vi "realTimeDisplay_AS2.vi"() -> ()   [LabVIEW 2016]
uses:
  <userlib>/RSA_API/RSA_API.lvlib
panel:
  in  "Done":bool
  in  "Cluster":T1 {"verticalUnit" items=["SpectrumVerticalUnit_dBm", "SpectrumVerticalUnit_Watt", "SpectrumVerticalUnit_Volt", "SpectrumVerticalUnit_Amp", "SpectrumVerticalUnit_dBmV"]; "window" items=["SpectrumWindow_Kaiser", "SpectrumWindow_Mil6dB", "SpectrumWindow_BlackmanHarris", "SpectrumWindow_Rectangle", "SpectrumWindow_FlatTop", "SpectrumWindow_Hann"]}
  in  "center freq":dbl
  in  "refLevel in":dbl
  in  "Trace number":u32(ring) items=["SpectrumTrace1", "SpectrumTrace2", "SpectrumTrace3"]
  out "traceData out":sgl[](graph)
  out "outTracePoints out":i32
  out "Trace Ready":bool
  out "enable out":bool
  out "refLevel out":dbl
  out "cf out":dbl
  in  "deviceID":i32
  out "deviceType out":string
  out "deviceSerial out":string
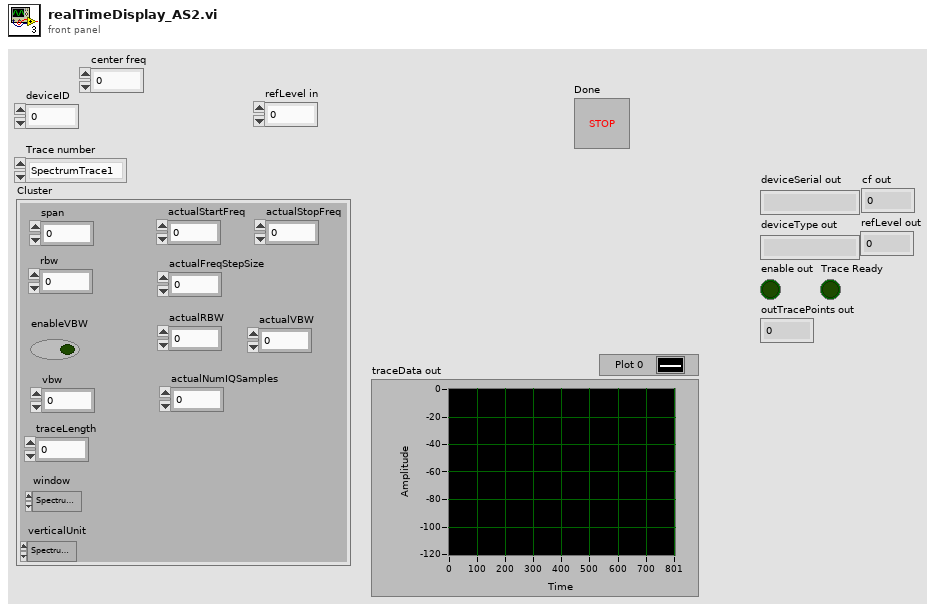
[diagram p1: front panel]
types:
  T1 = cluster{"span":dbl, "rbw":dbl, "enableVBW":bool, "vbw":dbl, "traceLength":i32, "window":u32, "verticalUnit":u32, "actualStartFreq":dbl, "actualStopFreq":dbl, "actualFreqStepSize":dbl, "actualRBW":dbl, "actualVBW":dbl, "actualNumIQSamples":i32}
  T2 = cluster{"span":dbl, "rbw":dbl, "enableVBW":bool, "vbw":dbl, "traceLength":i32, "window":u32, "verticalUnit":u32, dbl, dbl, "actualFreqStepSize":dbl, "actualRBW":dbl, "actualVBW":dbl, "actualNumIQSamples":i32}
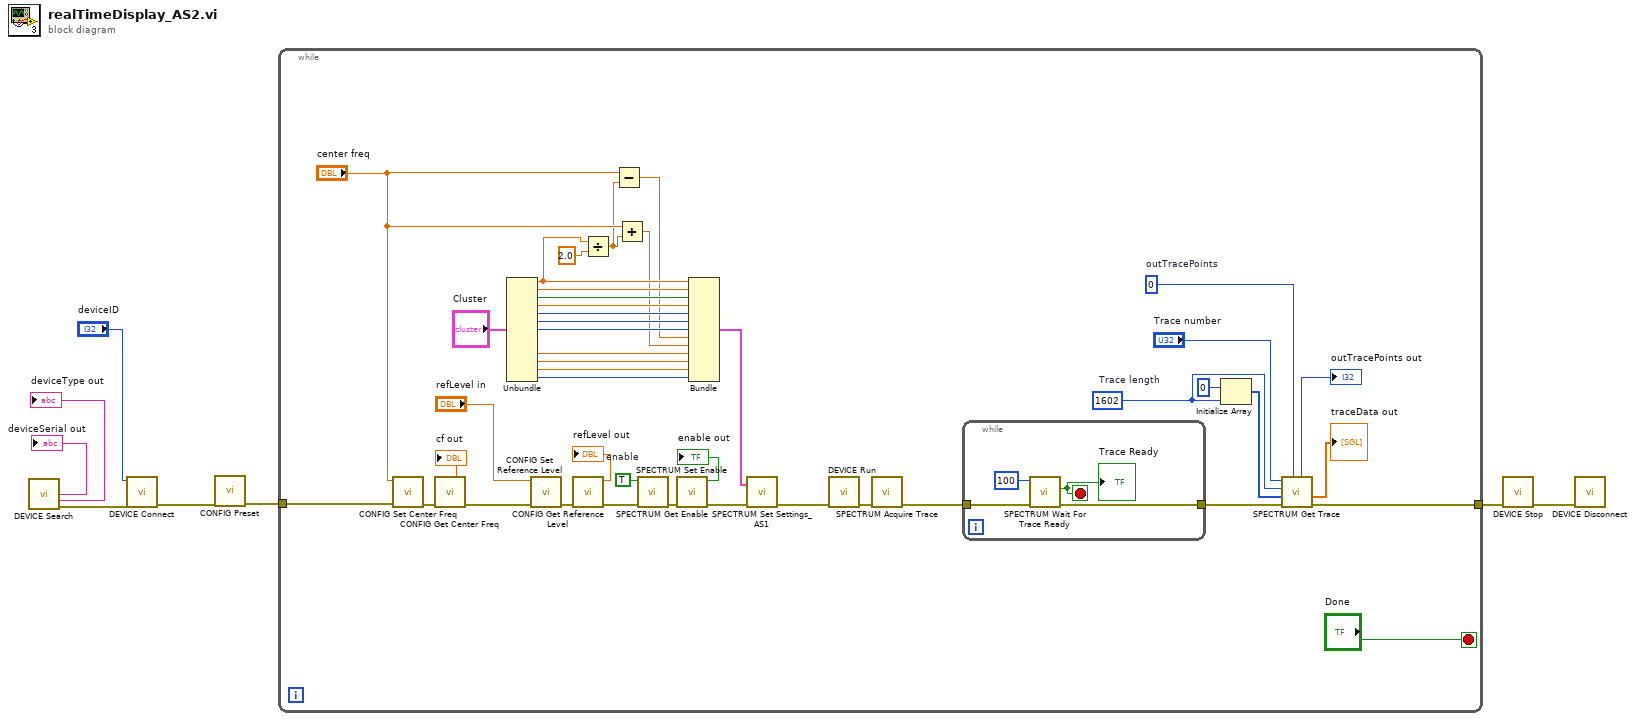
[diagram p0: block diagram]
diagram:
  n1 = call <userlib>:"DEVICE Search.vi"() -> ("deviceSerial out"=→"deviceSerial out":string, "deviceType out"=→"deviceType out":string, "error out"=w5:errorcluster)  [unwired: 10 in, 3 out]
  n2 = call <userlib>:"DEVICE Connect.vi"("error in (no error)"=w5, "deviceID"="deviceID") -> ("error out"=w4:errorcluster)  [unwired: 8 in, 1 out]
  n3 = call <userlib>:"CONFIG Preset.vi"("error in (no error)"=w4) -> ("error out"=w3:errorcluster)  [unwired: 9 in, 1 out]
  n4 = while {
    tunnel: w3 -> [w19]
    tunnel: [w29] -> w1
    stop <- "Done" stop-if-true
    w45 = TRUE  # enable
    w37 = 1602  # Trace length
    w38 = 0  # outTracePoints
    n5 = call <userlib>:"CONFIG Set Center Freq.vi"("error in (no error)"=w19, "cf"="center freq") -> ("error out"=w32:errorcluster)  [unwired: 8 in, 1 out]
    n6 = call <userlib>:"CONFIG Get Center Freq.vi"("error in (no error)"=w32) -> ("error out"=w51:errorcluster, "cf out"=→"cf out":dbl)  [unwired: 8 in, 1 out]
    n7 = Unbundle("Cluster") -> ("span"=w18:dbl, "rbw"=w26:dbl, "enableVBW"=w25:bool, "vbw"=w24:dbl, "traceLength"=w23:i32, "window"=w22:u32, "verticalUnit"=w21:u32, "actualFreqStepSize"=w14:dbl, "actualRBW"=w13:dbl, "actualVBW"=w12:dbl, "actualNumIQSamples"=w11:i32)  [unwired: 2 out]
    n8 = call <userlib>:"CONFIG Set Reference Level.vi"("error in (no error)"=w51, "refLevel"="refLevel in") -> ("error out"=w50:errorcluster)  [unwired: 8 in, 1 out]
    n9 = call <userlib>:"CONFIG Get Reference Level.vi"("error in (no error)"=w50) -> ("error out"=w46:errorcluster, "refLevel out"=→"refLevel out":dbl)  [unwired: 8 in, 1 out]
    n10 = Divide(x=w18, y=2.0) -> (x/y=w9:dbl)
    n11 = Subtract(x="center freq", y=w9) -> (x-y=w16:dbl)
    n12 = Add(x="center freq", y=w9) -> (x+y=w15:dbl)
    n13 = call <userlib>:"SPECTRUM Set Enable.vi"("error in (no error)"=w46, "enable"=w45) -> ("error out"=w44:errorcluster)  [unwired: 8 in, 1 out]
    n14 = call <userlib>:"SPECTRUM Get Enable.vi"("error in (no error)"=w44) -> ("error out"=w31:errorcluster, "enable out"=→"enable out":bool)  [unwired: 8 in, 1 out]
    n15 = Bundle("span"=w18, "rbw"=w26, "enableVBW"=w25, "vbw"=w24, "traceLength"=w23, "window"=w22, "verticalUnit"=w21, w16, w15, "actualFreqStepSize"=w14, "actualRBW"=w13, "actualVBW"=w12, "actualNumIQSamples"=w11) -> (w10:T2)  [unwired: 1 in]
    n16 = call "SPECTRUM Set Settings_AS1.vi"("error in (no error)"=w31, "Cluster"=w10) -> ("error out"=w28:errorcluster)  [unwired: 1 out]
    n17 = call <userlib>:"DEVICE Run.vi"("error in (no error)"=w28) -> ("error out"=w42:errorcluster)  [unwired: 9 in, 1 out]
    n18 = call <userlib>:"SPECTRUM Acquire Trace.vi"("error in (no error)"=w42) -> ("error out"=w41:errorcluster)  [unwired: 9 in, 1 out]
    n19 = while {
      tunnel: w41 -> [w53]
      tunnel: [w52] -> w40
      stop <- w54 stop-if-true
      n20 = call <userlib>:"SPECTRUM Wait For Trace Ready.vi"("error in (no error)"=w53, "timeoutMsec"=100) -> ("error out"=w52:errorcluster, "ready out"=w54:bool)  [unwired: 7 in, 1 out]
      "Trace Ready" <- w54
    }
    n21 = Initialize Array(0 ("element"), w37) -> (w35:i32[])
    n22 = call <userlib>:"SPECTRUM Get Trace.vi"("outTracePoints"=w38, "error in (no error)"=w40, "traceData"=w35, "maxTracePoints"=w37, "trace"="Trace number") -> ("error out"=w29:errorcluster, "traceData out"=→"traceData out":sgl[], "outTracePoints out"=→"outTracePoints out":i32)  [unwired: 3 in, 1 out]
  }
  n23 = call <userlib>:"DEVICE Stop.vi"("error in (no error)"=w1) -> ("error out"=w2:errorcluster)  [unwired: 9 in, 1 out]
  n24 = call <userlib>:"DEVICE Disconnect.vi"("error in (no error)"=w2) -> ()  [unwired: 9 in, 2 out]
